vi "Read On Board Memory (NVM).vi"(0 "Session Handle in":T1, 5 "Address":u16=171 format="%x", 11 "error in (no error)":errorcluster) -> (4 "Session Handle out":T1, 6 "Read Bytes":u8[](array[numeric]), 15 "error out":errorcluster)   [LabVIEW 2015, in "PAS.lvclass"]
uses:
  PAS.lvclass
  Typedefs/Session Handle.ctl
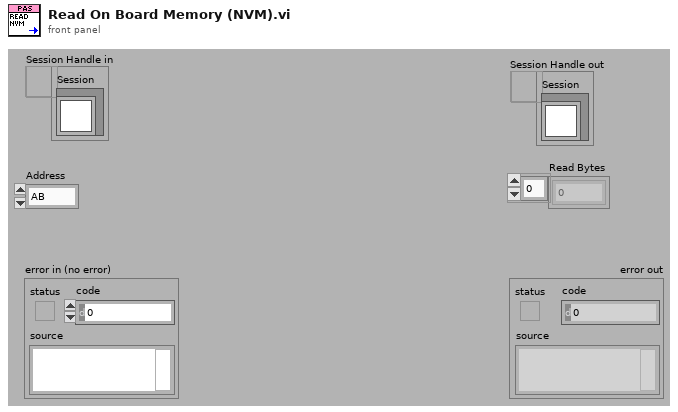
[diagram p1: front panel]
types:
  T1 = typedef "PAS.lvclass/Session Handle.ctl" = refnum<data-value>
  T2 = typedef "XNET Frame CAN.ctl" = cluster{"timestamp":timestamp, "payload":u8[], "identifier":u32, "type":T3, "extended?":bool, "echo?":bool}
  T3 = typedef "XNET Frame Type CAN.ctl" = u8
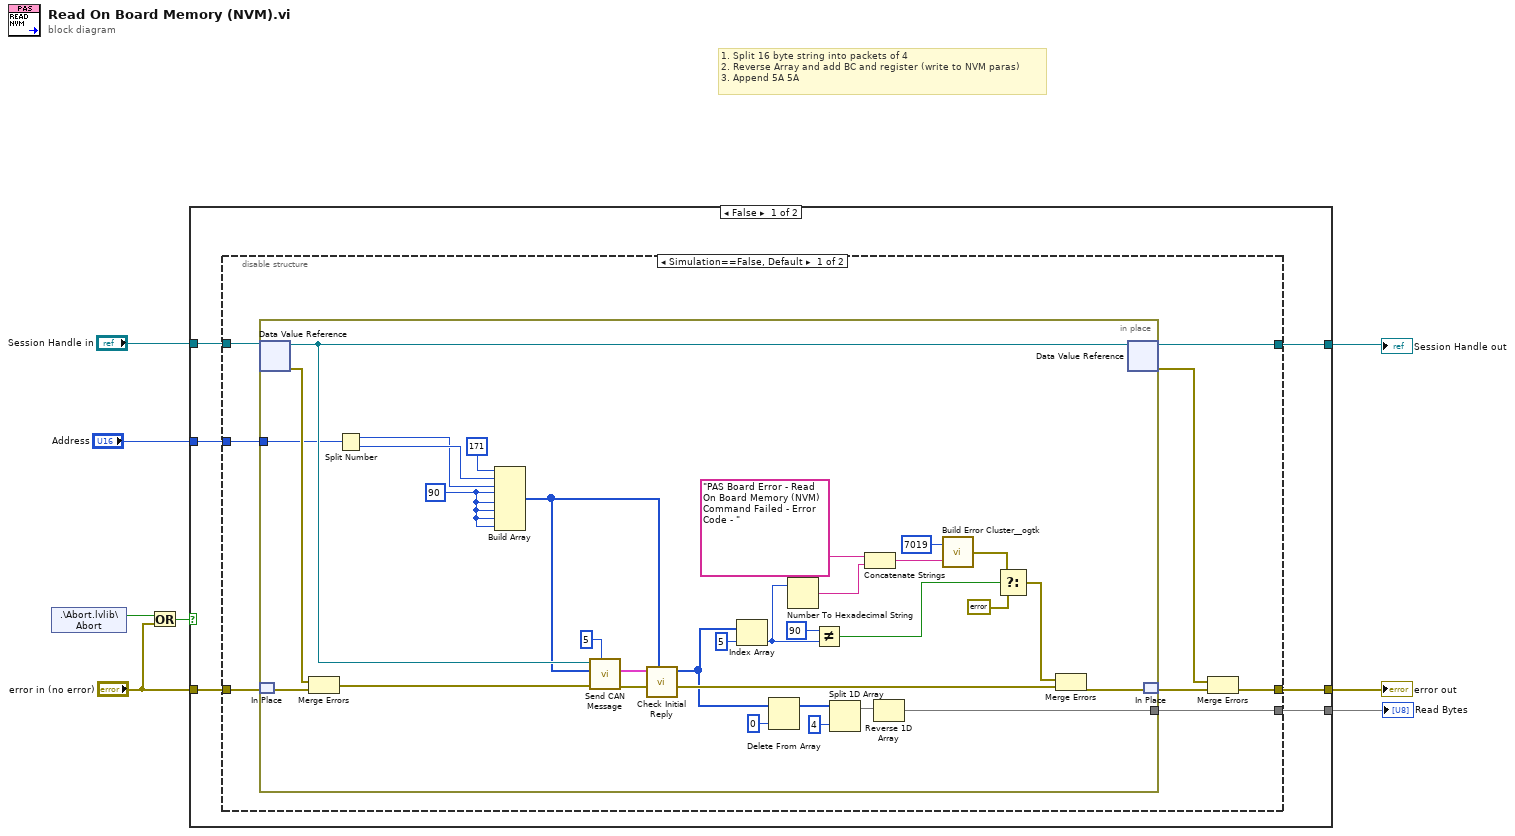
[diagram p0: block diagram]
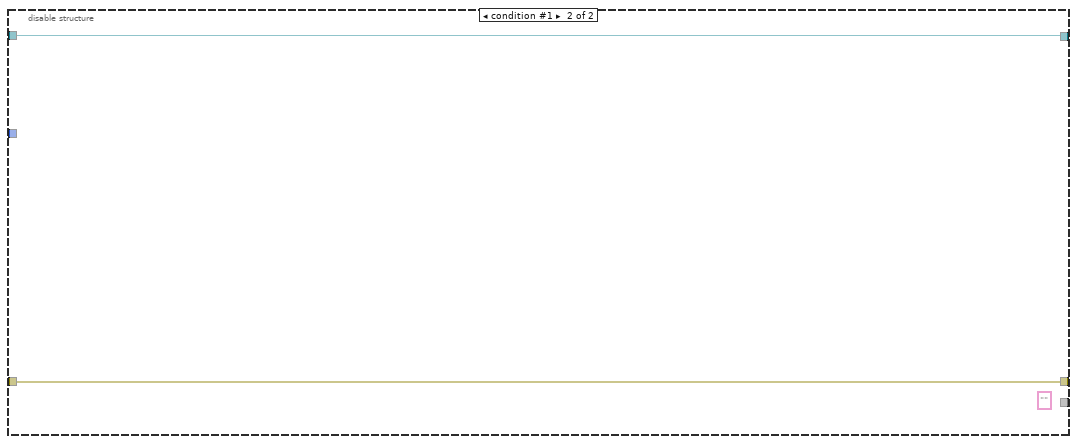
[diagram p2: hidden frame]
diagram:
  # "1. Split 16 byte string into packets of 4\n2. Reverse Array and add BC and register (write to NVM paras)\n3. Append 5A 5A"
  n1 = shared-variable ".\\Abort.lvlib\\Abort"() -> (w5:bool)  [unwired: 1 in, 1 out]
  n2 = Or(x=w5, y="error in (no error)") -> (x .or. y?=w3:bool)
  n3 = case shown="False" w3 {
    tunnel: [w14 w57] -> w7
    tunnel: [w13 w56] -> w6
    tunnel: "Session Handle in" -> [w12 w57]
    tunnel: "error in (no error)" -> [w11 w56]
    tunnel: "Address" -> [w10 _]
    tunnel: [w9 _] -> w1
    frame False {
      n4 = disable-structure shown="Simulation==False, Default" {
        disable-tunnel: [w22 w55] -> w14
        disable-tunnel: [w19 w54] -> w13
        disable-tunnel: w12 -> [w18 w55]
        disable-tunnel: w11 -> [w17 w54]
        disable-tunnel: w10 -> [w16 _]
        disable-tunnel: [w15 _] -> w9
        frame condition #0 (active) {
          n5 = in-place {
            in-place-border: w16 -> [w37]
            in-place-border: [w33] -> w15
            w34 = u8 90
            n6 = in-place-dvr #1(w18) -> (w50:refnum<class "PAS.lvclass">, w53:errorcluster)
            n7 = in-place-match #2(w17) -> (w52:errorcluster)
            n8 = Merge Errors(w53, w52) -> (w51:errorcluster)
            n9 = Split Number(x=w37) -> (hi(x)=w35:u8, lo(x)=w36:u8)
            n10 = Build Array(u8 171, w36, w35, w34, w34, w34, w34, w34) -> (w45:u8[])
            n11 = call "Send CAN Message.vi"("Number of Retries"=5, "error in (no error)"=w51, "payload"=w45, "Gas In"=w50) -> ("error out"=w41:errorcluster, "Reply"=w46:T2[])  [unwired: 5 in, 1 out]
            n12 = call "Check Initial Reply.vi"("Write Message"=w45, "Reply"=w46) -> ("Data Packet"=w23:u8[])  [unwired: 7 in, 2 out]
            n13 = Index Array(array=w23, index=5) -> (element=w29:u8)
            n14 = Delete From Array(array=w23, index=0) -> (array with subset deleted=w24:u8[])  [unwired: 1 in, 1 out]
            n15 = Number To Hexadecimal String(2:w29) -> (0:w28:string)  [unwired: 1 in]
            n16 = Not Equal?(x=u8 90, y=w29) -> (x != y?=w26:bool)
            n17 = Split 1D Array(array=w24, index=4) -> (first subarray=w38:u8[])  [unwired: 1 out]
            n18 = Concatenate Strings("PAS Board Error - Read On Board Memory (NVM) Command Failed - Error Code - " ("string"), w28) -> (w27:string)
            n19 = Reverse 1D Array(array=w38) -> (reversed array=w33:u8[])
            n20 = call <userlib>:"Build Error Cluster__ogtk.vi"("String to Prepend to source (\"\")"=w27, "code"=7019) -> ("error out"=w43:errorcluster)
            n21 = Select(t=w43, s=w26, f=errorcluster {"status"=FALSE, "code"=0, "source"=""}) -> (s? t:f=w40:errorcluster)
            n22 = Merge Errors(w40, w41) -> (w49:errorcluster)
            n23 = in-place-dvr #1(w50) -> (w22:T1, w20:errorcluster)
            n24 = in-place-match #2(w49) -> (w21:errorcluster)
          }
          n25 = Merge Errors(w20, w21) -> (w19:errorcluster)
        }
        frame condition #1 {
          (unwired) "" ("string")
        }
      }
    }
    frame True {
    }
  }
  "Session Handle out" <- w7
  "error out" <- w6
  "Read Bytes" <- w1
